vi "Initialize Default.vi"(8 "error in (no error)":errorcluster, 11 "Core Threads Configuration in":refnum<class "Thread Configuration.lvclass">) -> (0 "error out":errorcluster, 3 "Core Threads Configuration out":refnum<class "Thread Configuration.lvclass">)   [LabVIEW 2020, in "DSF Core.lvlib" / "Thread Configuration.lvclass"]
uses:
  Thread Configuration.lvclass
  Typedefs/Core Thread Configuration.ctl
  Thread Configuration.lvclass/Thread Configuration.ctl
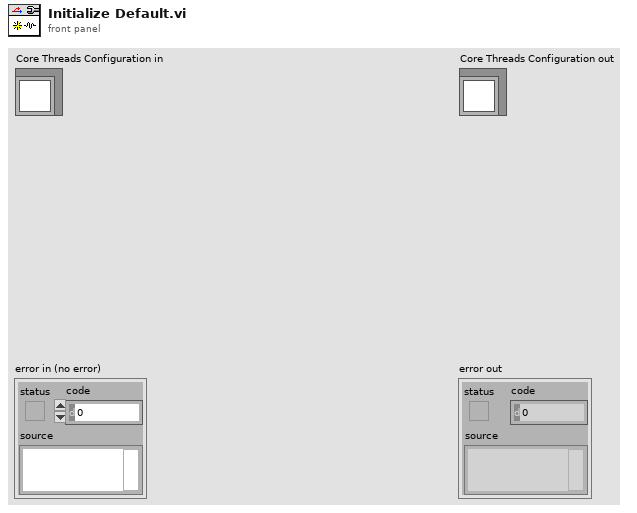
[diagram p1: front panel]
types:
  T1 = typedef "DSF Core.lvlib/Thread Configuration.lvclass/Core Thread Configuration.ctl" = cluster{"processor":i32, "priority offset":i16}
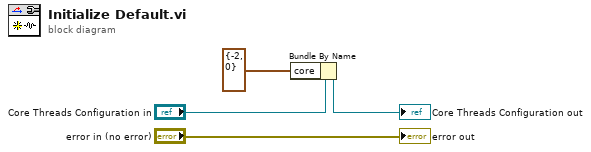
[diagram p0: block diagram]
diagram:
  n1 = Bundle By Name(cluster="Core Threads Configuration in", "core"=T1 {"processor"=-2, "priority offset"=0} ("configuration")) -> (→"Core Threads Configuration out":refnum<class "Thread Configuration.lvclass">)
  "error out" <- "error in (no error)"
